vi "JGP3.vi"() -> ()   [LabVIEW 2019]
doc: "This VI explores while loops, shift registers, and the quotient and remainder (modulus) tool for every index we get the sum of the previous value and of the current value for ex 1+2 =3 then 3+3=6...\n\nJuan Gamez\nP3600\nCSUSB Physics"
panel:
  out "sum":i32
  in  "stop early":bool
  out "divisible by 5":bool
  out "loop index":i32
  # "Juan Gamez\nP3600"
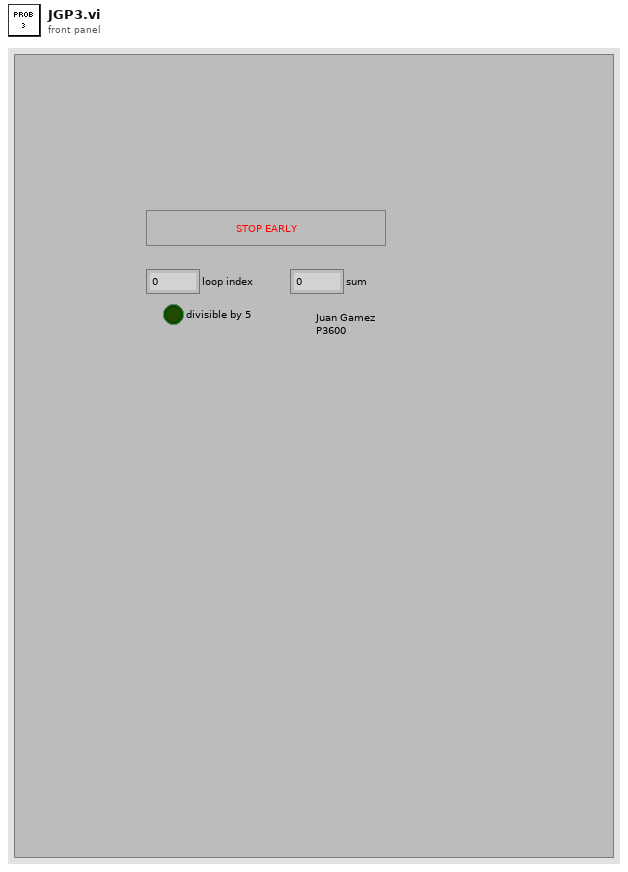
[diagram p1: front panel]
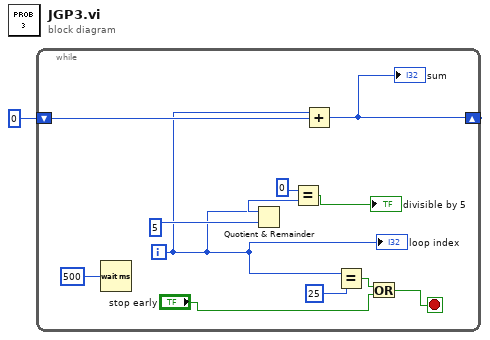
[diagram p0: block diagram]
diagram:
  n1 = while {
    shift-right: [w2] -> _
    shift-left: 0 -> [w4]
    i -> [w3]
    stop <- w12 stop-if-true
    n2 = Wait (ms)(milliseconds to wait=u32 500) -> ()  [unwired: 1 out]
    n3 = Quotient & Remainder(x=w3, y=5) -> (x-y*floor(x/y)=w8:i32)  [unwired: 1 out]
    n4 = Equal?(x=0, y=w8) -> (x = y?=→"divisible by 5":bool)
    n5 = Add(x=w3, y=w4) -> (x+y=w2:i32)
    "sum" <- w2
    n6 = Equal?(x=w3, y=25) -> (x = y?=w11:bool)
    n7 = Or(x=w11, y="stop early") -> (x .or. y?=w12:bool)
    "loop index" <- w3
  }
